vi "Read Arguments.vi"(8 "error in (no error)":errorcluster, 11 "ParsedData in":refnum<class "ParsedData.lvclass">) -> (0 "error out":errorcluster, 2 "Arguments":T1, 3 "ParsedData out":refnum<class "ParsedData.lvclass">)   [LabVIEW 2022 SP3, in "ArgumentParser.lvlib" / "ParsedData.lvclass"]
uses:
  ParsedData.lvclass
  ParsedData.lvclass/ParsedData.ctl
  _Arguments.ctl
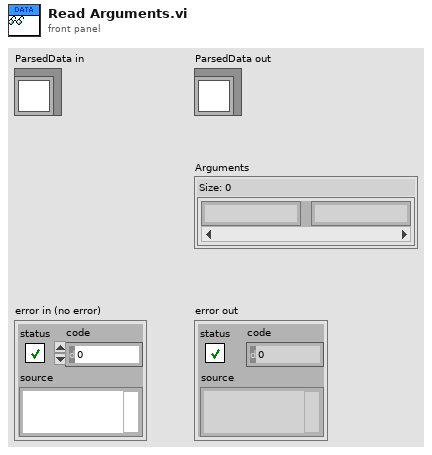
[diagram p1: front panel]
types:
  T1 = typedef "ArgumentParser.lvlib/ParsedData.lvclass/_Arguments.ctl" = map{string, string}
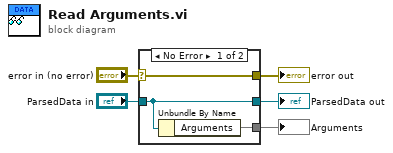
[diagram p0: block diagram]
diagram:
  n1 = case shown="No Error" "error in (no error)" {
    selector: "error in (no error)" -> [w8 w9]
    tunnel: [w8 w9] -> w4
    tunnel: [w7 w10] -> w2
    tunnel: "ParsedData in" -> [w7 w10]
    tunnel: [w6 _] -> w1
    frame No Error {
      n2 = Unbundle By Name(w7) -> ("Arguments"=w6:T1)
    }
    frame Error {
    }
  }
  "error out" <- w4
  "ParsedData out" <- w2
  "Arguments" <- w1
